vi "CAN Get Status.vi"(9 "pCANStatus":T1, 10 "CANIndex":u8, 11 "DevHandle":i32) -> (1 "pCANStatus out":T1, 3 "function return":i32)   [LabVIEW 2010, in "usb2can.lvlib"]
doc: "int WINAPI CAN_GetStatus(int DevHandle, unsigned char CANIndex, PCAN_STATUS pCANStatus);"
uses:
  usb2can.lvlib
  USB2XXX.dll
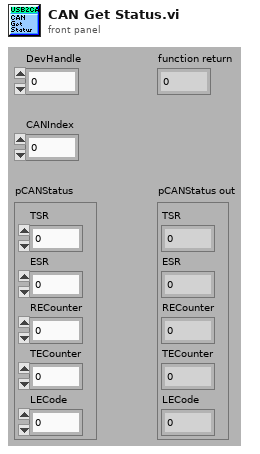
[diagram p1: front panel]
types:
  T1 = cluster{"TSR":u32, "ESR":u32, "RECounter":u8, "TECounter":u8, "LECode":u8}
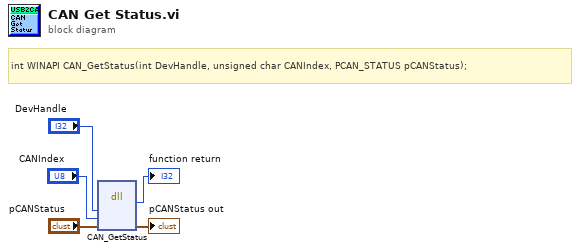
[diagram p0: block diagram]
diagram:
  # "int WINAPI CAN_GetStatus(int DevHandle, unsigned char CANIndex, PCAN_STATUS pCANStatus);"
  n1 = dll-call lib="G:/OtherWork/USB2XXX_Example/trunk/Labview/PublicFiles/USB2XXX.*" fn="CAN_GetStatus"("DevHandle"="DevHandle", "CANIndex"="CANIndex", "pCANStatus"="pCANStatus") -> (→"function return":i32, "pCANStatus"=→"pCANStatus out":T1)  [unwired: 5 in, 2 out]
